vi "serial_test(1).vi"() -> ()   [LabVIEW 2017]
doc: "This example performs writes and reads on a serial port, as directed by the user. You can press the Write and Read buttons, and change the Read Count, while the example is running.\n\nThe parameters set for the serial port must match the parameters of the connected instrument or device. In this example, the Read Count parameter specifies the number of bytes that the serial port reads. If there were more bytes at the port than the specified number, those bytes would not be read. If there were less bytes at the port than the specified number, you would receive a timeout error.\n\nThis example expands upon the flow control options for XON and XOFF, allowing the user to choose those control characters. Also, the user can enable or disable a termination character. Some devices require a termination character in order to identify the end of command strings. Some devices send a termination character to signify the end of data to be read. This example shows how you can end the Read operation once a termination character is detected in the buffer and/or append a termination character at the end of the Write data."
uses:
  Program Files (x86)/National Instruments/LabVIEW 2017/examples/Instrument IO/Serial/support/Serial - Settings.ctl
  Program Files (x86)/National Instruments/LabVIEW 2017/examples/Instrument IO/Serial/support/Serial - XON-XOFF Characters.ctl
  Program Files (x86)/National Instruments/LabVIEW 2017/examples/Instrument IO/Serial/support/Serial - ASCII Characters.ctl
  <vilib>/Instr/_visa.llb/VISA Configure Serial Port (Instr).vi
panel:
  out "배열":string[](array[string])
  out "연결된 문자열":string
  out "부분 문자열":string
  out "원소":string
  out "웨이브폼 그래프":dbl[](graph)
  out "출력 배열":dbl[](array[numeric])
  out "숫자":dbl
  in  "Termination Character":u8=10 format="%.0x"
  in  "End Write on Termination Character?":bool=TRUE
  in  "Stop":bool
  in  "Command":string="*IDN?"
  in  "Read Count":u32=1000
  out "Response":string
  in  "Write":bool
  in  "Read":bool
  in  "XON/XOFF Characters":T1={"XON"=enum."DC1", "XOFF"=enum."DC3"}
  in  "Serial Settings":T3={"baud rate"=9600, "data bits"=8, "parity"=enum."None", "stop bits"=10, "flow control"=0} {"flow control" items=["None"=0, "XON/XOFF"=1, "RTS/CTS"=2, "DTR/DSR"=4]; "stop bits" items=["1.0"=10, "1.5"=15, "2.0"=20]; "data bits" min=5 max=8 step=1; "baud rate" items=["75"=75, "110"=110, "134"=134, "150"=150, "300"=300, "600"=600, "1200"=1200, "1800"=1800, "2400"=2400, "4800"=4800, "7200"=7200, "9600"=9600, "14400"=14400, "19200"=19200, "28800"=28800, "38400"=38400, "56000"=56000, "57600"=57600, "115200"=115200, "128000"=128000, "230400"=230400]}
  in  "End Read on Termination Character?":bool=TRUE
  in  "VISA resource name":refnum<visa-resource-name>="COM1"
  # "Overview: Demonstrates the use of the VISA functions to write commands to and read responses from a serial instrument continuously in a loop.\nRequirements: NI-VISA Driver\nInstructions:\n1. Run the VI.\n2. Specify a Command and click the Write button.\n3. Read a Response by clicking the Read button.\n4. Click Stop to stop the VI."
  # "0xA is equivalent to a '\\n' character, which is a line feed."
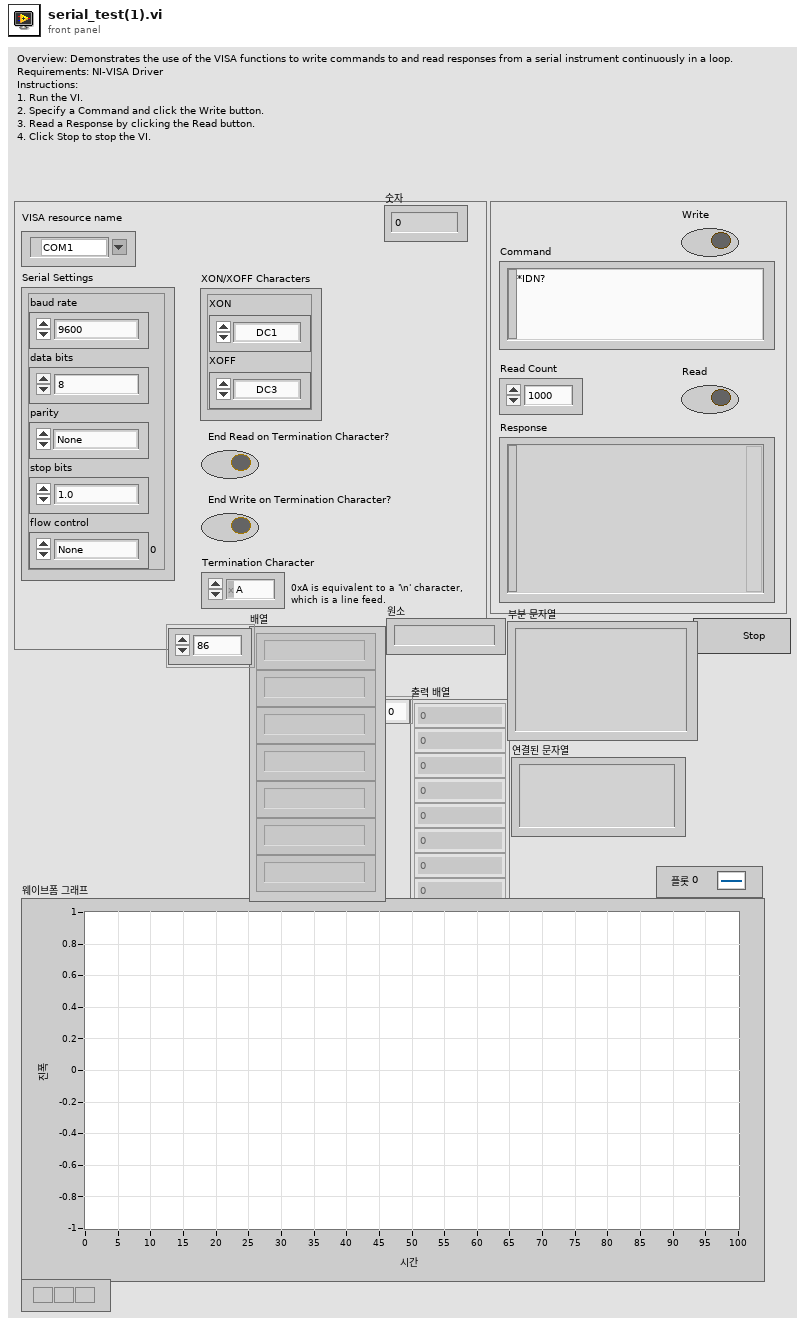
[diagram p1: front panel]
types:
  T1 = typedef "Serial - XON-XOFF Characters.ctl" = cluster{"XON":T2, "XOFF":T2}
  T2 = typedef "Serial - ASCII Characters.ctl" = enum16{"NUL", "SOH", "STX", "ETX", "EOT", "ENQ", "ACK", "BEL", "BS", "HT", "LF", "VT", "FF", "CR", "SO", "SI", "DLE", "DC1", "DC2", "DC3", "DC4", "NAK", "SYN", "ETB", "CAN", "EM", "SUB", "ESC", "FS", "GS", "RS", "US", "SP", "!", "\"", "#", "$", "%", "&", "'", "(", ")", "*", "+", ",", "- (-)", ".", "/", "0", "1", "2", "3", "4", "5", "6", "7", "8", "9", ":", ";", "<", "=", ">", "?", "@", "A", "B", "C", "D", "E", "F", "G", "H", "I", "J", "K", "L", "M", "N", "O", "P", "Q", "R", "S", "T", "U", "V", "W", "X", "Y", "Z", "[", "\\", "]", "^", "_", "`", "a", "b", "c", "d", "e", "f", "g", "h", "i", "j", "k", "l", "m", "n", "o", "p", "q", "r", "s", "t", "u", "v", "w", "x", "y", "z", "{", "|", "}", "~"}
  T3 = typedef "Serial - Settings.ctl" = cluster{"baud rate":u32, "data bits":u16, "parity":enum16{"None", "Odd", "Even", "Mark", "Space"}, "stop bits":u16, "flow control":u16}
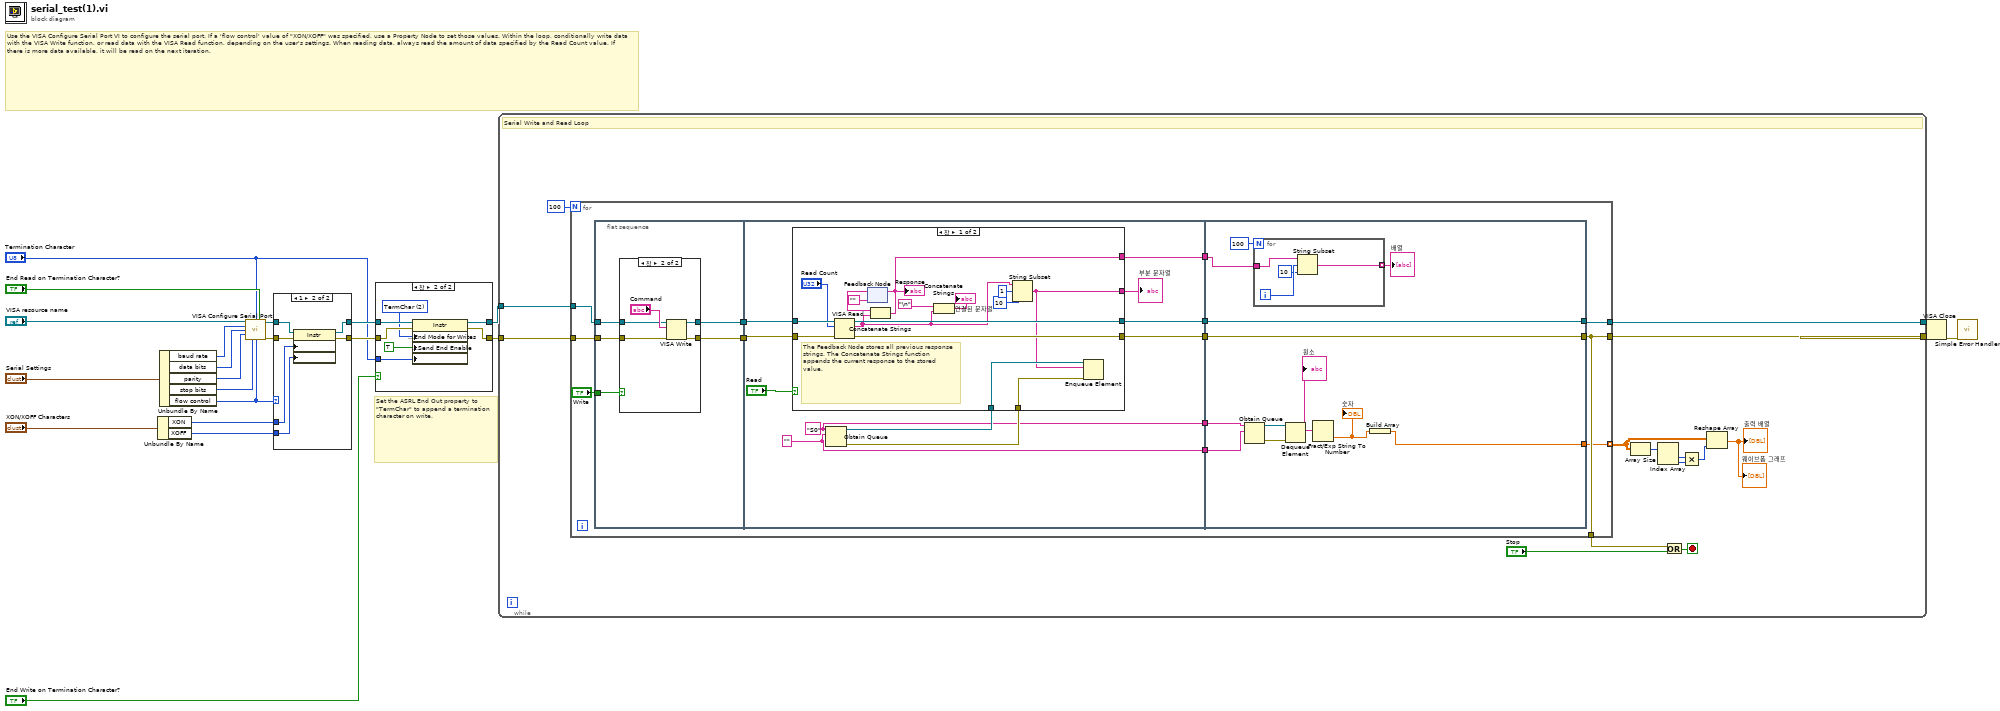
[diagram p0: block diagram]
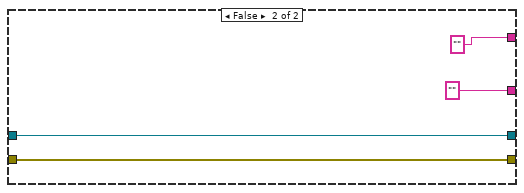
[diagram p5: hidden frame]
diagram:
  # "Set the ASRL End Out property to \"TermChar\" to append a termination character on write."
  # "Use the VISA Configure Serial Port VI to configure the serial port. If a 'flow control' value of \"XON/XOFF\" was specified, use a Property Node to set those values. Within the loop, conditionally write data with the VISA Write function, or read data with the VISA Read function, depending on the user's settings. When reading data, always read the amount of data specified by the Read Count value. If there is more data available, it will be read on the next iteration."
  n1 = Unbundle By Name("XON/XOFF Characters") -> ("XON"=w10:T2, "XOFF"=w9:T2)
  n2 = Unbundle By Name("Serial Settings") -> ("baud rate"=w15:u32, "data bits"=w16:u16, "parity"=w17:enum16{"None", "Odd", "Even", "Mark", "Space"}, "stop bits"=w18:u16, "flow control"=w11:u16)
  n3 = call-poly "VISA Configure Serial Port"("VISA resource name"="VISA resource name", "termination char\n(0xA = '\\n' = LF)"="Termination Character", "Enable Termination\nChar (T)"="End Read on Termination Character?", "baud rate (9600)"=w15, "data bits (8)"=w16, "parity (0:none)"=w17, "stop bits (10: 1 bit)"=w18, "flow control (0:none)"=w11) -> ("VISA resource name out"=w19:refnum<visa-resource-name>, "error out"=w20:errorcluster)  [unwired: 2 in, 4 out]
  n4 = case shown="1" w11 {
    tunnel: [w23 w30] -> w8
    tunnel: [w24 w29] -> w6
    tunnel: w20 -> [w23 w28]
    tunnel: w19 -> [w24 w27]
    tunnel: w10 -> [_ w26]
    tunnel: w9 -> [_ w25]
    frame Default {
    }
    frame 1 {
      n5 = property class="Instr"(reference=w27, error in=w28, "Serial Settings:Flow Control XON Character"=w26, "Serial Settings:Flow Control XOFF Character"=w25) -> (reference out=w29:refnum<visa-resource-name>, error out=w30:errorcluster)
    }
  }
  n6 = case shown="참" "End Write on Termination Character?" {
    tunnel: w6 -> [w31 w39]
    tunnel: w8 -> [w32 w38]
    tunnel: [w31 w37] -> w3
    tunnel: [w32 w36] -> w7
    tunnel: "Termination Character" -> [_ w34]
    frame False {
    }
    frame True {
      w35 = u16 2 items=["None", "LastBit", "TermChar", "Break"] ("Serial Settings:Serial End Mode for Writes")
      n7 = property class="Instr"(reference=w39, error in=w38, "Serial Settings:End Mode for Writes"=w35, "Message Based Settings:Send End Enable"=TRUE, "Message Based Settings:Termination Character"=w34) -> (reference out=w37:refnum<visa-resource-name>, error out=w36:errorcluster)
    }
  }
  n8 = while {
    tunnel: w7 -> [w51]
    tunnel: w3 -> [w50]
    tunnel: [w48] -> w2
    tunnel: [w47] -> w1
    stop <- w53 stop-if-true
    # "Serial Write and Read Loop"
    n9 = for {
      N: 100 -> [_]
      tunnel: w51 -> [w59]
      tunnel: w50 -> [w58]
      tunnel: [w56] -> w49
      tunnel: [w57] -> w48
      tunnel: [w56] -> w47
      tunnel: [w55] -> w41 mode=indexing
      n10 = flat-sequence {
        tunnel: w58 -> [w71]
        tunnel: w59 -> [w70]
        tunnel: "Write" -> [w67]
        tunnel: [w69] -> w66
        tunnel: [w68] -> w65
        tunnel: w66 -> [w86]
        tunnel: w65 -> [w85]
        tunnel: [w88] -> w64
        tunnel: [w87] -> w63
        tunnel: [w82] -> w62
        tunnel: [w81] -> w61
        tunnel: [w79] -> w54
        tunnel: [w120] -> w56
        tunnel: [w121] -> w57
        tunnel: w64 -> [w121]
        tunnel: w63 -> [w120]
        tunnel: w62 -> [w119]
        tunnel: w61 -> [w118]
        tunnel: [w114] -> w55
        tunnel: w54 -> [w110]
        frame #0 {
          n11 = case shown="참" w67 {
            tunnel: w71 -> [w73 w77]
            tunnel: w70 -> [w72 w76]
            tunnel: [w73 w75] -> w69
            tunnel: [w72 w74] -> w68
            frame False {
            }
            frame True {
              n12 = VISA Write(VISA resource name=w77, write buffer="Command", error in (no error)=w76) -> (VISA resource name out=w75:refnum<visa-resource-name>, error out=w74:errorcluster)  [unwired: 1 out]
            }
          }
        }
        frame #1 {
          w81 = ""
          w82 = "S0" ("이름(이름없음)")
          n13 = Obtain Queue(name (unnamed)=w82, element data type=w81) -> (queue out=w84:refnum<queue>, error out=w83:errorcluster)  [unwired: 3 in, 1 out]
          n14 = case shown="참" "Read" {
            tunnel: [w103 w109] -> w88
            tunnel: w86 -> [w105 w109]
            tunnel: [w101 w108] -> w87
            tunnel: w85 -> [w104 w108]
            tunnel: w84 -> [w100 _]
            tunnel: w83 -> [w99 _]
            tunnel: [w96 ""] -> w80
            tunnel: [w90 ""] -> w79
            frame True {
              # "The Feedback Node stores all previous response strings. The Concatenate Strings function appends the current response to the stored value."
              n15 = VISA Read(VISA resource name=w105, byte count="Read Count", error in (no error)=w104) -> (VISA resource name out=w103:refnum<visa-resource-name>, read buffer=w91:string, error out=w101:errorcluster)  [unwired: 1 out]
              n16 = feedback #1("") -> (w98:string)
              n17 = Concatenate Strings(w98, w91) -> (w90:string)
              "Response" <- w90
              n18 = feedback-in #1(w90) -> ()
              n19 = Concatenate Strings("\n", w91) -> (→"연결된 문자열":string)
              n20 = String Subset(string=w91, offset (0)=1 ("오프셋(0)"), length (rest)=10 ("길이(나머지)")) -> (substring=w96:string)
              n21 = Enqueue Element(queue=w100, element=w96, error in (no error)=w99) -> ()  [unwired: 1 in, 3 out]
            }
            frame False {
            }
          }
          "부분 문자열" <- w80
        }
        frame #2 {
          n22 = Obtain Queue(name (unnamed)=w119, element data type=w118) -> (queue out=w117:refnum<queue>, error out=w116:errorcluster)  [unwired: 3 in, 1 out]
          n23 = for {
            N: 100 -> [_]
            tunnel: w110 -> [w123]
            tunnel: [w122] -> w112 mode=indexing
            i -> [w125]
            n24 = String Subset(string=w123, offset (0)=w125, length (rest)=10 ("길이(나머지)")) -> (substring=w122:string)
          }
          "배열" <- w112
          n25 = Dequeue Element(queue=w117, error in (no error)=w116) -> (element=w111:string)  [unwired: 1 in, 3 out]
          "원소" <- w111
          n26 = Fract/Exp String To Number(string=w111) -> (number=w115:dbl)  [unwired: 3 in, 1 out]
          "숫자" <- w115
          n27 = Build Array(w115) -> (w114:dbl[])
        }
      }
    }
    n28 = Array Size(array=w41) -> (size(s)=w44:i32[])
    n29 = Index Array(array=w44) -> (element #1=w43:i32, element #2=w42:i32)  [unwired: 2 in]
    n30 = Or(x=w49, y="Stop") -> (x .or. y?=w53:bool)
    n31 = Multiply(x=w43, y=w42) -> (x*y=w45:i32)
    n32 = Reshape Array(w41, w45) -> (→"출력 배열" →"웨이브폼 그래프":dbl[])
  }
  n33 = VISA Close(VISA resource name=w2, error in (no error)=w1) -> (error out=w12:errorcluster)
  n34 = call <vilib>:"Simple Error Handler.vi"("error in (no error)"=w12) -> ()  [unwired: 1 in, 8 out]
